vi "Integrate.vi"(11 "New samples in":u64) -> (0 "Next Sample":u8, 3 "Sum out":u16)   [LabVIEW 2012]
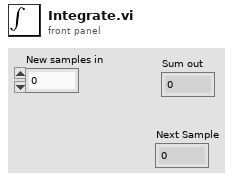
[diagram p1: front panel]
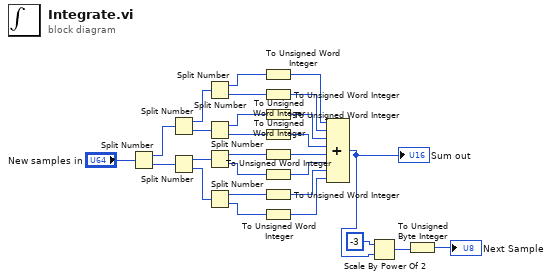
[diagram p0: block diagram]
diagram:
  n1 = Split Number(x="New samples in") -> (hi(x)=w26:u32, lo(x)=w25:u32)
  n2 = Split Number(x=w26) -> (hi(x)=w24:u16, lo(x)=w23:u16)
  n3 = Split Number(x=w25) -> (hi(x)=w22:u16, lo(x)=w21:u16)
  n4 = Split Number(x=w24) -> (hi(x)=w20:u8, lo(x)=w19:u8)
  n5 = Split Number(x=w23) -> (hi(x)=w18:u8, lo(x)=w17:u8)
  n6 = Split Number(x=w22) -> (hi(x)=w16:u8, lo(x)=w15:u8)
  n7 = Split Number(x=w21) -> (hi(x)=w14:u8, lo(x)=w13:u8)
  n8 = To Unsigned Word Integer(number=w20) -> (unsigned 16bit integer=w12:u16)
  n9 = To Unsigned Word Integer(number=w19) -> (unsigned 16bit integer=w11:u16)
  n10 = To Unsigned Word Integer(number=w18) -> (unsigned 16bit integer=w10:u16)
  n11 = To Unsigned Word Integer(number=w17) -> (unsigned 16bit integer=w9:u16)
  n12 = To Unsigned Word Integer(number=w16) -> (unsigned 16bit integer=w8:u16)
  n13 = To Unsigned Word Integer(number=w15) -> (unsigned 16bit integer=w7:u16)
  n14 = To Unsigned Word Integer(number=w14) -> (unsigned 16bit integer=w6:u16)
  n15 = To Unsigned Word Integer(number=w13) -> (unsigned 16bit integer=w5:u16)
  n16 = Compound Arithmetic op=ADD(w12, w11, w10, w9, w8, w7, w6, w5) -> (w3:u16)
  "Sum out" <- w3
  n17 = Scale By Power Of 2(n=i16 -3, x=w3) -> (x*2^n=w2:u16)
  n18 = To Unsigned Byte Integer(number=w2) -> (unsigned 8bit integer=→"Next Sample":u8)
